vi "SUB_GET_MAC_USNID.vi"(0 "URL":string, 1 "Stage":string, 2 "SN":string, 3 "ID_TYPE":u8, 4 "Sequence":i16) -> (5 "output param":string)   [LabVIEW 2011]
uses:
  data/MCSDLL.dll
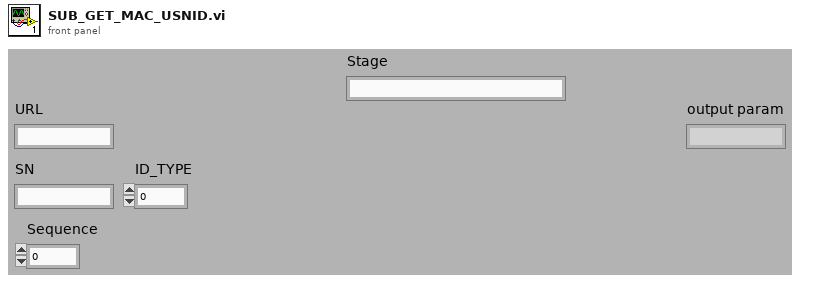
[diagram p1: front panel]
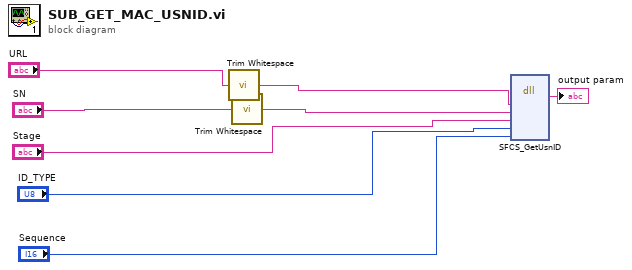
[diagram p0: block diagram]
diagram:
  n1 = call <vilib>:"Trim Whitespace.vi"("string"="URL") -> ("trimmed string"=w5:string)  [unwired: 1 in]
  n2 = call <vilib>:"Trim Whitespace.vi"("string"="SN") -> ("trimmed string"=w2:string)  [unwired: 1 in]
  n3 = dll-call lib="D:/S8300E_Project/data/MCSDLL.dll" fn="SFCS_GetUsnID"("URL"=w5, "SN"=w2, "Stage"="Stage", "ID_TYPE"="ID_TYPE", "Sequence"="Sequence") -> (→"output param":string)  [unwired: 8 in, 2 out]
